vi "Actor Core.vi"(8 "error in":errorcluster, 11 "RandomDataChart in":refnum<class "NumericCounter.lvclass">) -> (0 "error out":errorcluster, 3 "Actor out":refnum<class "Actor.lvclass">)   [LabVIEW 2015, in "TestViewables.lvlib" / "NumericCounter.lvclass"]
doc: "(<B>Filename</B>: Actor Framework.lvlib:Actor.lvclass:Actor Core.vi)\n\nReceives messages to the actor, reacts to them, and initiates any error handling that may shut the actor down.\n\nDescendant classes may override this VI to append parallel tasks for the actor to complete while it handles messages. Overrides use the Call Parent Method node.\n\n<License>\nCopyright © 2017 Composed Systems, LLC | All rights reserved\nwww.composed.io\n\nAuthor: Ethan Stern <ethan.stern@composed.io>\n\nThis software is provided \"AS IS\" WITHOUT WARRANTIES, either express or implied, AND IS FOR EDUCATIONAL PURPOSES ONLY.\n</License>"
uses:
  NumericCounter.lvclass
  <vilib>/ActorFramework/Actor/Actor.lvclass
  Framework/IViewable/IViewable/IViewable.lvclass
  Framework/IObserver/IObserver/IObserver.lvclass
panel:
  out "Bound Model Data":dbl caption="Random Number"
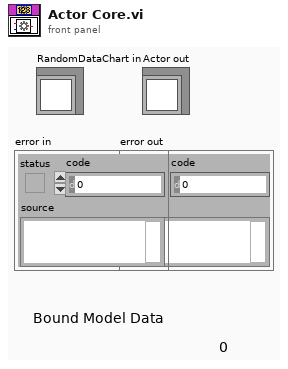
[diagram p1: front panel]
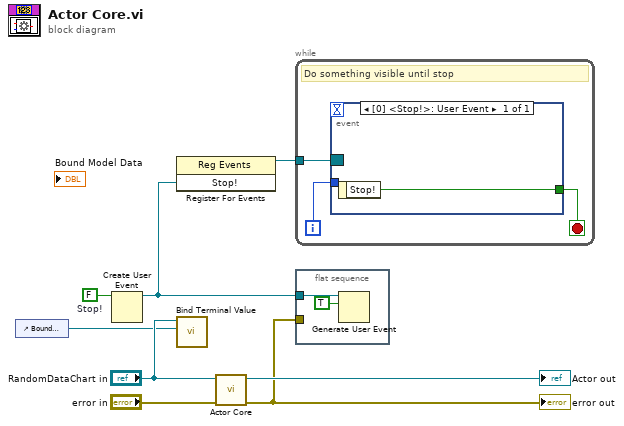
[diagram p0: block diagram]
diagram:
  w6 = FALSE  # Stop!
  n1 = control-ref of="Bound Model Data"() -> (w1:refnum<vi>)
  n2 = Create User Event(user event datatype=w6) -> (user event=w3:refnum<user-event>)  [unwired: 1 in, 1 out]
  n3 = register-events(w3) -> (reference out=w4:refnum<event-registration>)  [unwired: 2 in, 1 out]
  n4 = call "Bind Terminal Value.vi"("Ctl Refnum"=w1, "IObserver in"="RandomDataChart in") -> ()  [unwired: 8 in, 2 out]
  n5 = call-parent "Actor Core.vi"("error in"="error in", "IViewable In"="RandomDataChart in") -> ("error out"=w5:errorcluster, "Actor out"=→"Actor out":refnum<class "Actor.lvclass">)  [unwired: 8 in]
  "error out" <- w5
  n6 = while {
    tunnel: w4 -> [w11]
    i -> [w9]
    stop <- w10 stop-if-true
    # "Do something visible until stop"
    n7 = event shown="[0] <Stop!>: User Event" {
      selector: w11 -> [_]
      dyn-events: _ -> [_]
      timeout: _ -> [_]
      tunnel: [w12] -> w10
      tunnel: w9 -> [_]
      event User Event {
        n8 = event-data() -> ("Stop!"=w12:bool)  [unwired: 1 in]
      }
    }
  }
  n9 = flat-sequence {
    tunnel: w3 -> [w14]
    tunnel: w5 -> [_]
    frame #0 {
      n10 = Generate User Event(user event=w14, event data cluster=TRUE ("event data")) -> ()  [unwired: 2 in, 2 out]
    }
  }
